vi "SimpleLiveAppWithROI.vi"() -> ()   [LabVIEW 2018]
uses:
  C:/Users/Public/Documents/Photometrics/PMQI-LabViewSamples/Examples/Dependencies/PVCamNET.dll
  Public/Documents/Photometrics/PMQI-LabViewSamples/Examples/Dependencies/PVCamNET.dll
panel:
  in  "Full CCD":bool
  in  "Full CCD Height":u16
  in  "Full CCD Width":u16
  in  "Get ROI":bool
  in  "Height":u16
  in  "Y":u16
  in  "Width":u16
  in  "X":u16
  in  "Exposure Time":dbl
  in  "Live":bool
  in  "Camera Status":bool
  in  "Uninit":bool
  in  "Live stop":bool
  in  "Live start":bool
  in  "Init":bool
  # "SimpleLiveAppWithROI.vi\n\nDescription:\nThis sample code lets the user use live mode in an event driven structure.\nThe user can create a ROI from CamWindow and find out the coordinate.\n\nSteps to run:\n1. Click \"Run\"\n2. Click \"Open\"\n3. Enter Exposure Time\n4. Click \"Live start\"\n5. Click \"Live stop\"\n6. Right click on CamWindow and add a ROI.\n7. Click \"Get ROI\"\n8. Click \"Live start\"\n9. Click \"Live stop\"\n10. Right click on CamWindow and delete a ROI.\n11. Click \"Close\""
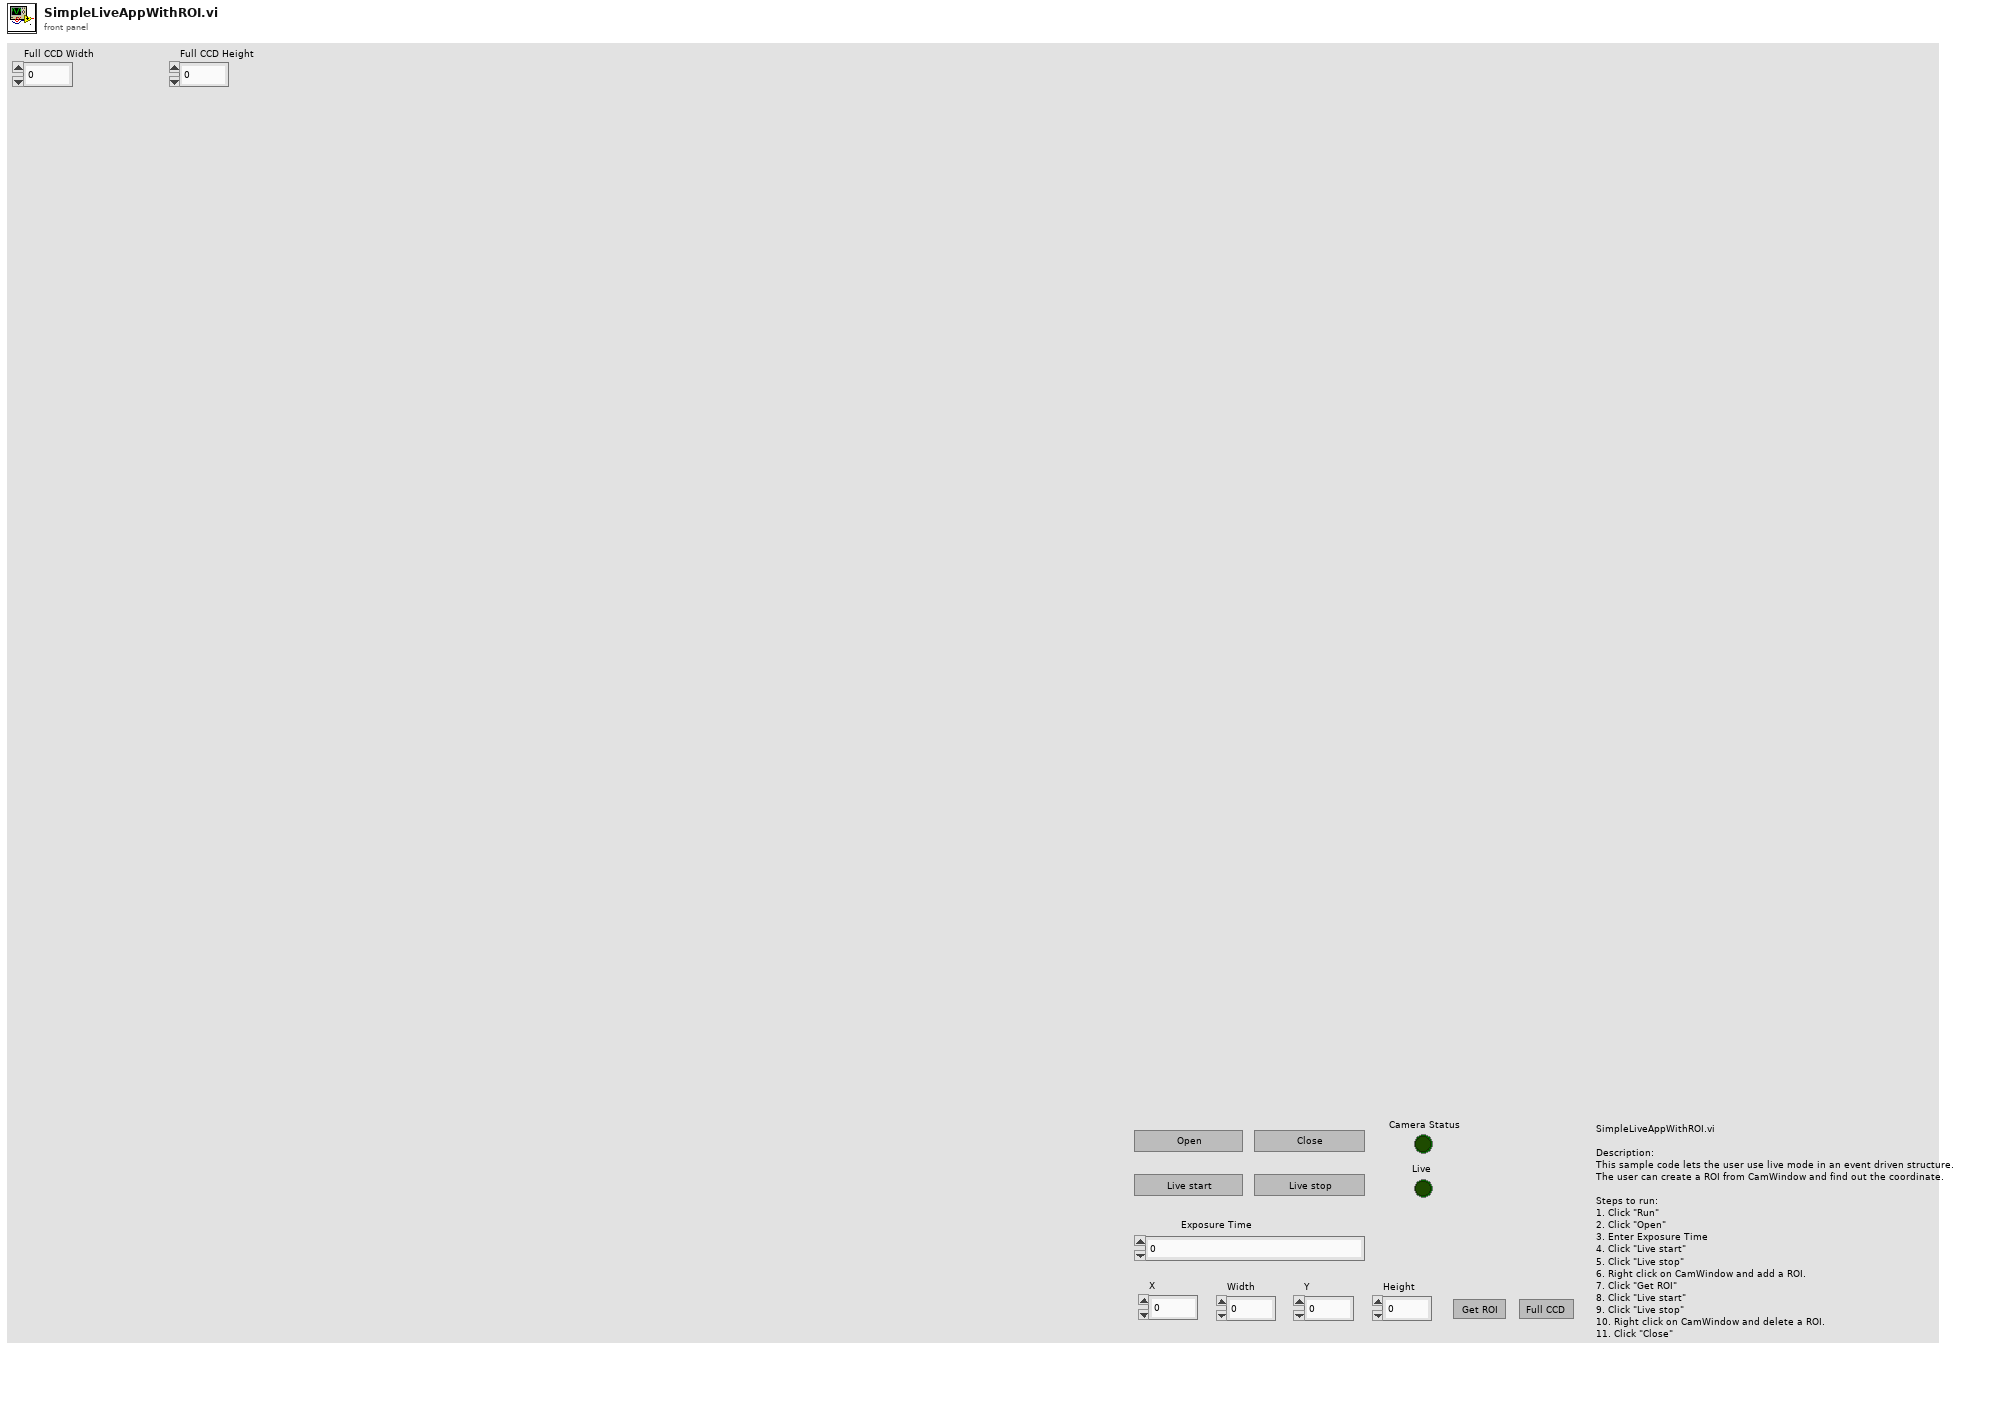
[diagram p1: front panel]
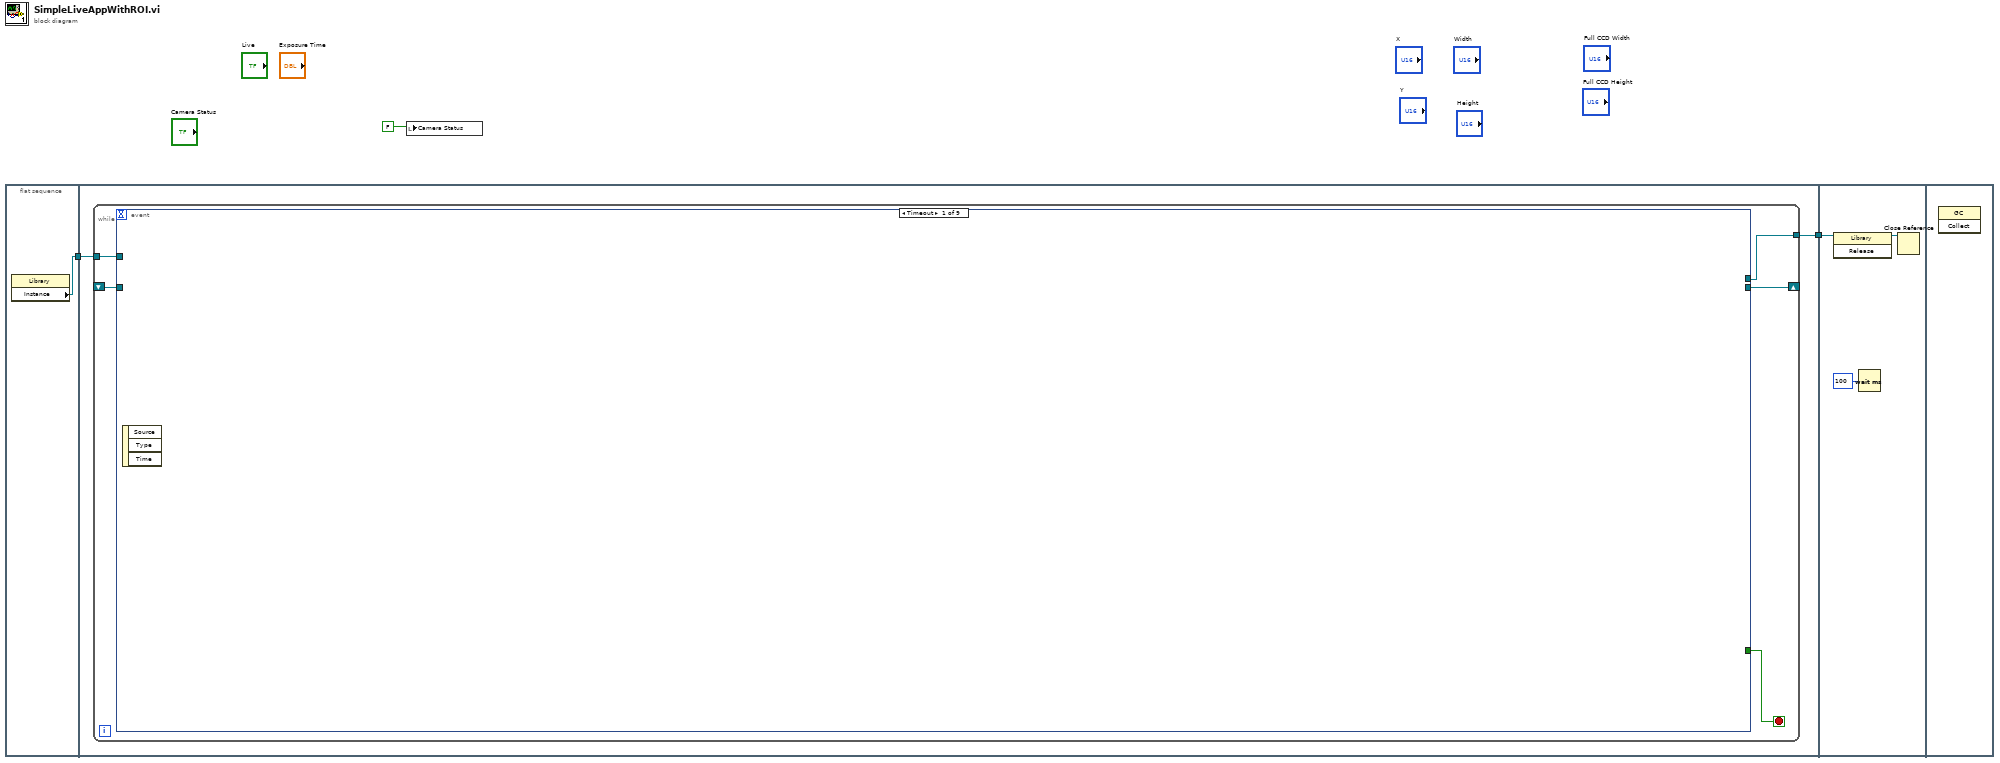
[diagram p0: block diagram]
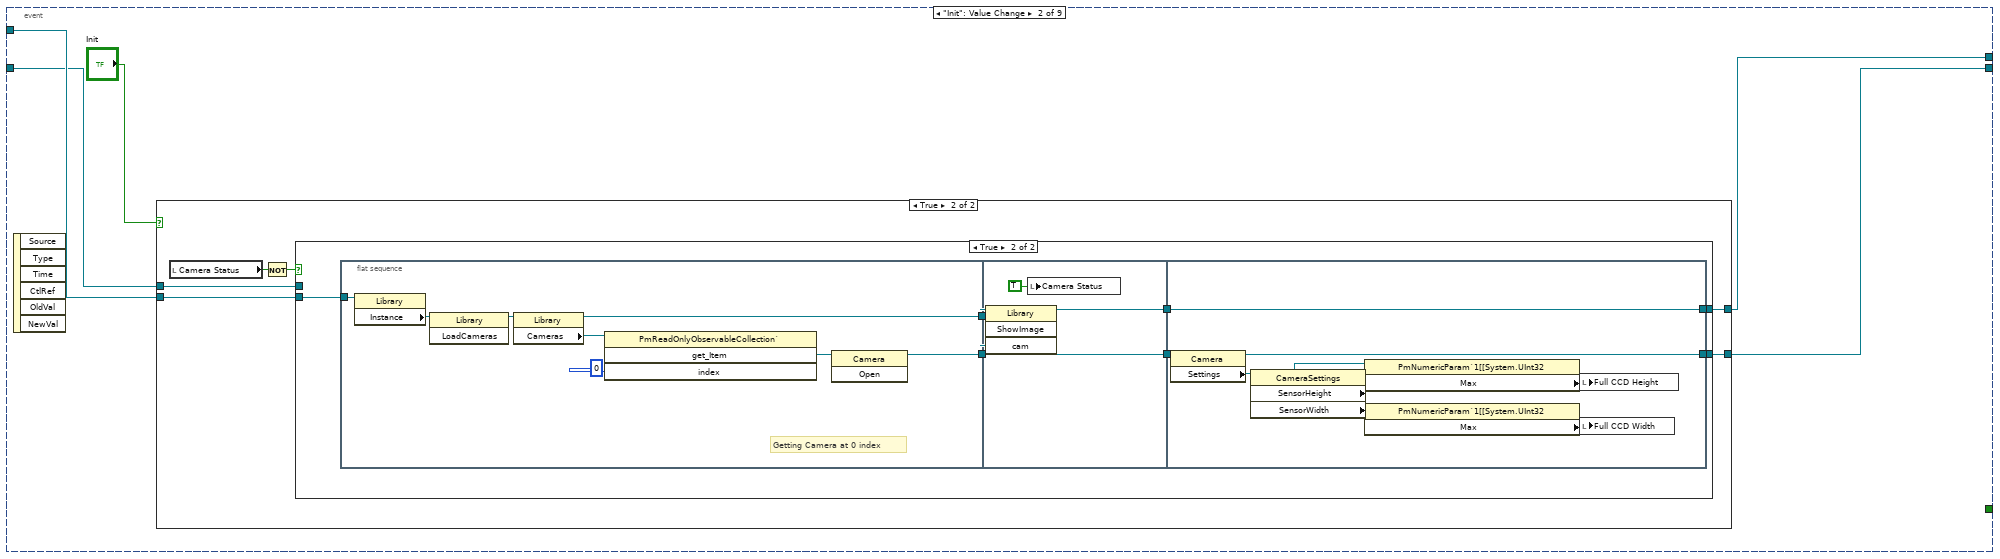
[diagram p2: hidden frame]
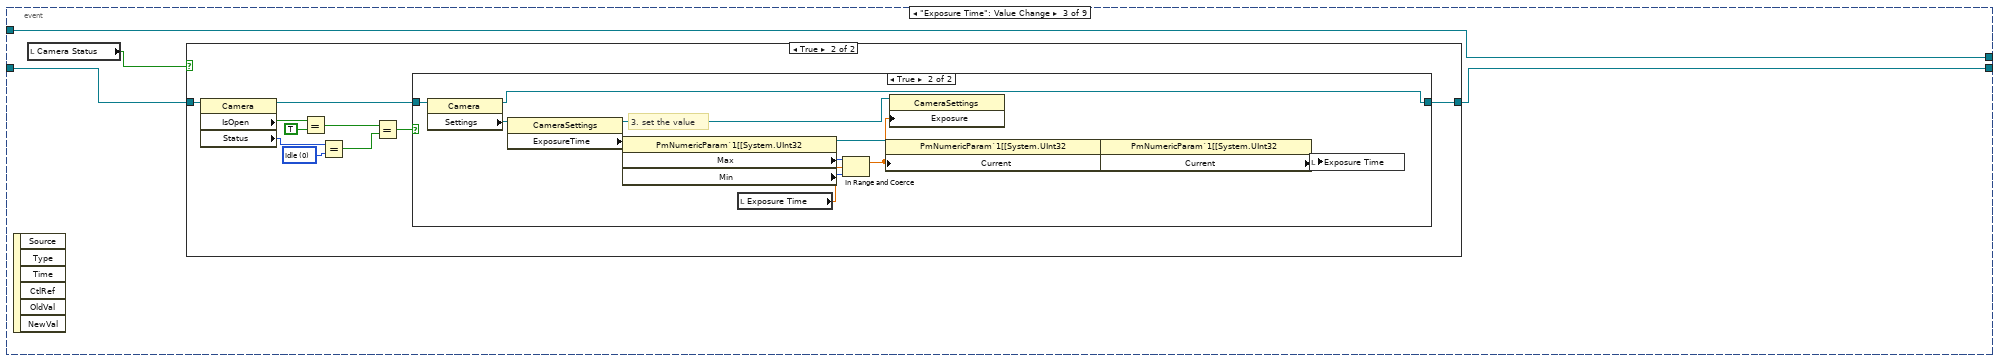
[diagram p5: hidden frame]
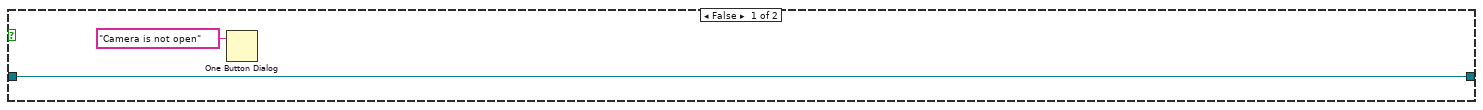
[diagram p6: hidden frame]
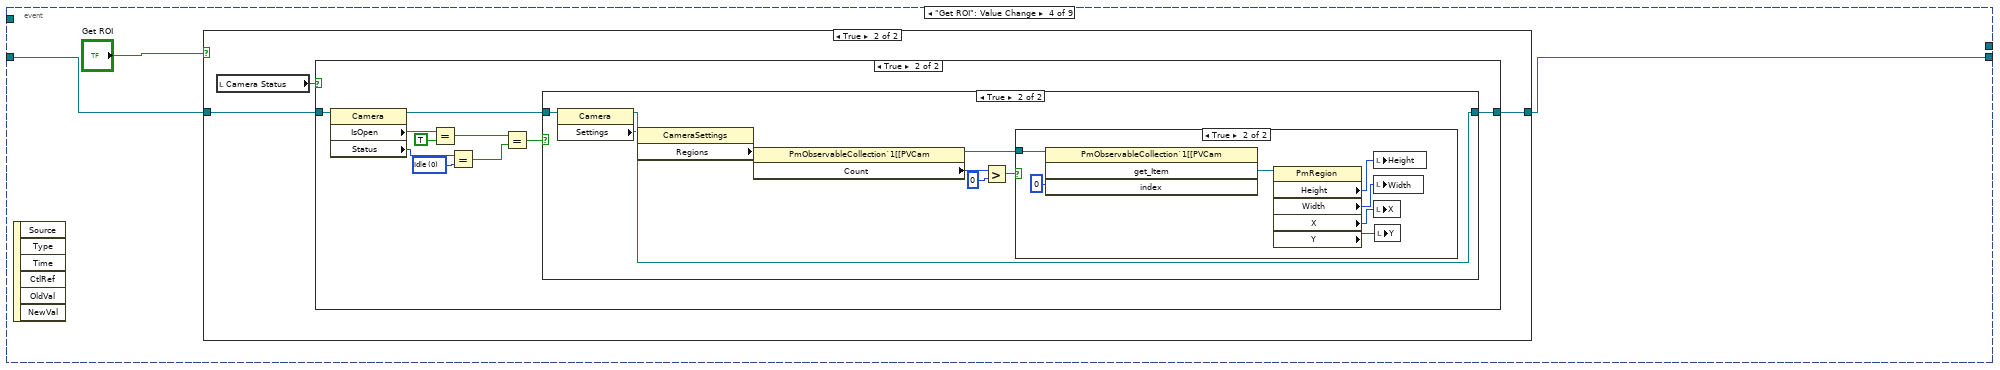
[diagram p8: hidden frame]
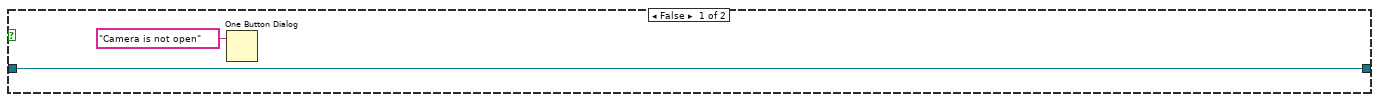
[diagram p10: hidden frame]
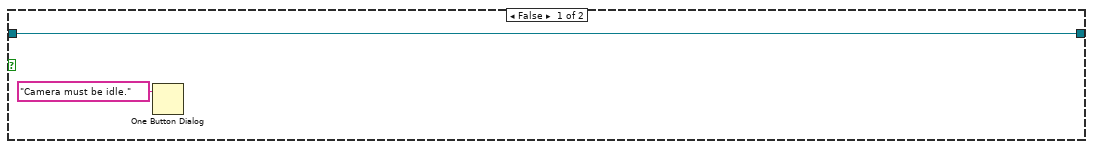
[diagram p11: hidden frame]
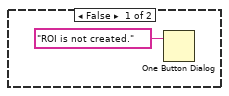
[diagram p12: hidden frame]
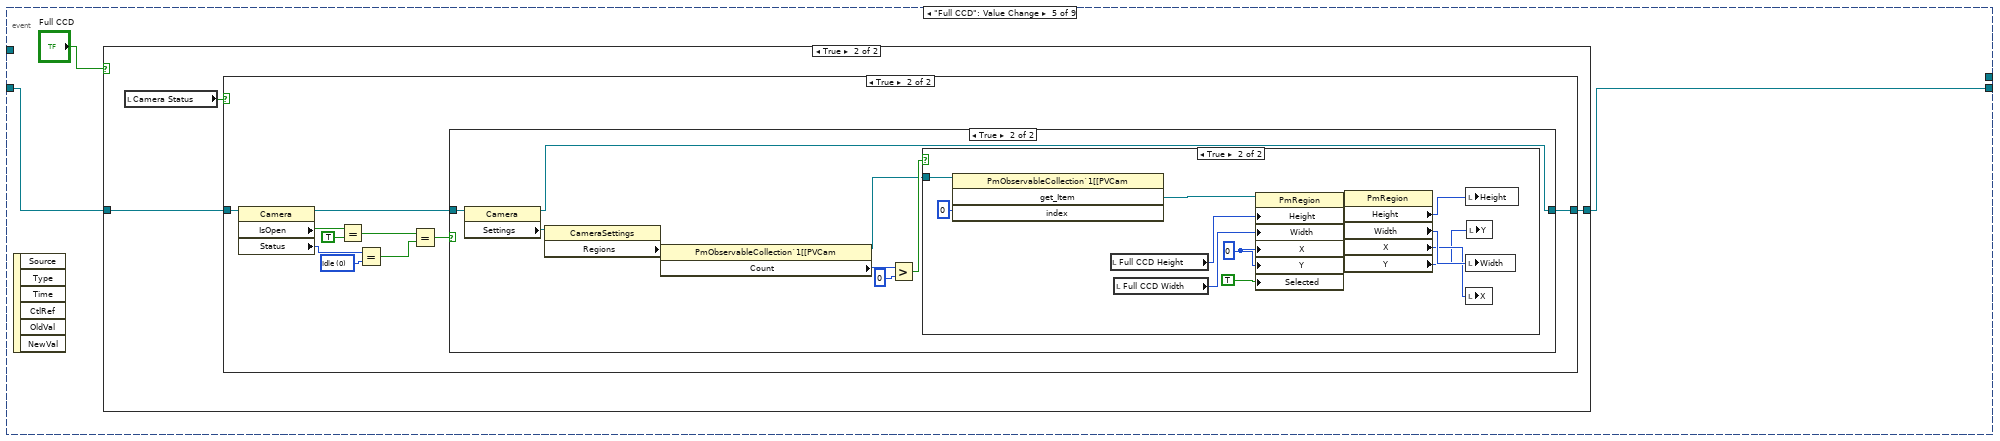
[diagram p13: hidden frame]
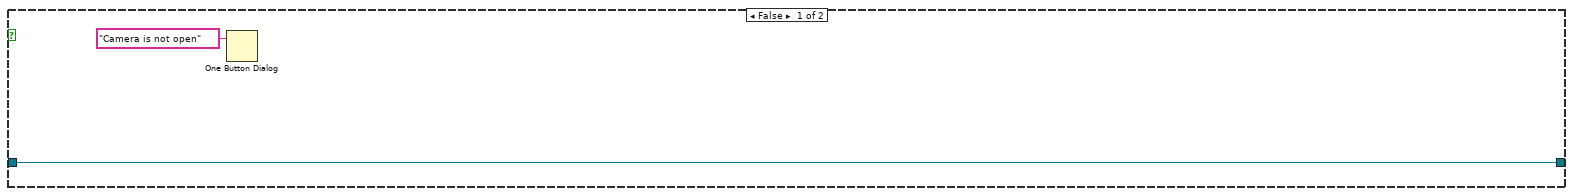
[diagram p15: hidden frame]
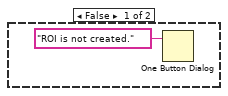
[diagram p17: hidden frame]
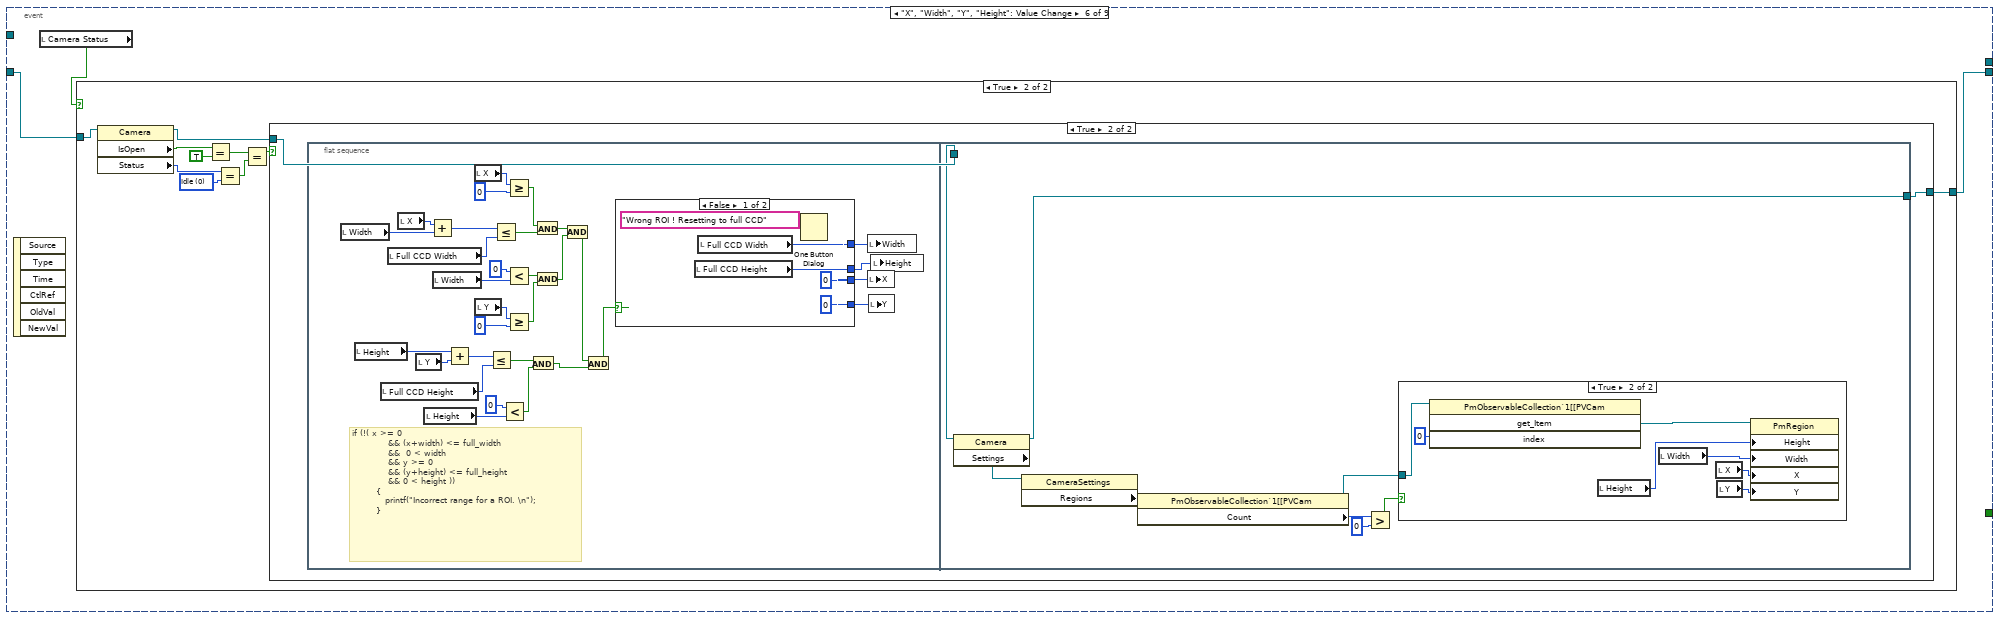
[diagram p18: hidden frame]
diagram:
  n1 = flat-sequence {
    tunnel: [w4] -> w3
    tunnel: w3 -> [w6]
    tunnel: [w5] -> w2
    tunnel: w2 -> [w317]
    frame #0 {
      n2 = property class="Library"() -> ("Instance"=w4:refnum<k24>)  [unwired: 2 in, 2 out]
    }
    frame #1 {
      n3 = while {
        tunnel: w6 -> [w11]
        shift-right: [w7] -> _
        shift-left: _ -> [w9]
        tunnel: [w10] -> w5
        stop <- w8 stop-if-true
        n4 = event shown="[0] Timeout" {
          selector: _ -> [_ _ _ _ _ _ _ _ _]
          dyn-events: _ -> [_ _ _ _ _ _ _ _ _]
          timeout: _ -> [_ _ _ _ _ _ _ _ _]
          tunnel: w11 -> [_ w16 w54 _ _ _ w234 _ w289]
          tunnel: [_ w15 w56 w83 w121 w162 w235 w264 w290] -> w7
          tunnel: [_ w14 w54 _ _ _ w234 _ w289] -> w10
          tunnel: w9 -> [_ w13 w57 w85 w122 w161 w236 w265 w291]
          tunnel: [_ _ _ _ _ _ _ _ w288] -> w8
          event Timeout {
            n5 = event-data() -> ()  [unwired: 1 in, 3 out]
          }
          event "Init": Value Change {
            n6 = event-data() -> ()  [unwired: 1 in, 6 out]
            n7 = case shown="True" "Init" {
              tunnel: w16 -> [w18 w24]
              tunnel: [w17 w23] -> w15
              tunnel: [w18 w22] -> w14
              tunnel: w13 -> [w17 w19]
              frame False {
              }
              frame True {
                n8 = local read "Camera Status"() -> (w21:bool)
                n9 = Not(x=w21) -> (.not. x?=w20:bool)
                n10 = case shown="True" w20 {
                  tunnel: w24 -> [w25 w31]
                  tunnel: [w26 w30] -> w23
                  tunnel: [w25 w29] -> w22
                  tunnel: w19 -> [w26 _]
                  frame False {
                  }
                  frame True {
                    n11 = flat-sequence {
                      tunnel: w31 -> [w36]
                      tunnel: [w38] -> w33
                      tunnel: [w37] -> w32
                      tunnel: w33 -> [w44]
                      tunnel: w32 -> [w45]
                      tunnel: [w45] -> w28
                      tunnel: [w43] -> w27
                      tunnel: [w53] -> w29
                      tunnel: [w48] -> w30
                      tunnel: w28 -> [w52]
                      tunnel: w27 -> [w53]
                      frame #0 {
                        # "Getting Camera at 0 index"
                        n12 = property class="Library"(reference=w36) -> ("Instance"=w35:refnum<k24>)  [unwired: 1 in, 2 out]
                        n13 = invoke class="Library" method="LoadCameras"(reference=w35) -> (reference out=w34:refnum<k24>)  [unwired: 2 in, 2 out]
                        n14 = property class="Library"(reference=w34) -> (reference out=w38:refnum<k24>, "Cameras"=w41:refnum<k24>)  [unwired: 1 in, 1 out]
                        n15 = invoke class="PmReadOnlyObservableCollection`" method="get_Item"(reference=w41, "index"=0) -> ("get_Item"=w39:refnum<k24>)  [unwired: 2 in, 3 out]
                        n16 = invoke class="Camera" method="Open"(reference=w39) -> (reference out=w37:refnum<k24>)  [unwired: 2 in, 2 out]
                      }
                      frame #1 {
                        n17 = invoke class="Library" method="ShowImage"(reference=w44, "cam"=w45) -> (reference out=w43:refnum<k24>)  [unwired: 2 in, 3 out]
                        n18 = local write "Camera Status"(TRUE ("Camera Status")) -> ()
                      }
                      frame #2 {
                        n19 = property class="Camera"(reference=w52) -> (reference out=w48:refnum<k24>, "Settings"=w51:refnum<k24>)  [unwired: 1 in, 1 out]
                        n20 = property class="CameraSettings"(reference=w51) -> ("SensorHeight"=w50:refnum<k24>, "SensorWidth"=w49:refnum<k24>)  [unwired: 1 in, 2 out]
                        n21 = property class="PmNumericParam`1[[System.UInt32"(reference=w50) -> ("Max"=w47:u32)  [unwired: 1 in, 2 out]
                        n22 = property class="PmNumericParam`1[[System.UInt32"(reference=w49) -> ("Max"=w46:u32)  [unwired: 1 in, 2 out]
                        n23 = local write "Full CCD Height"(w47) -> ()
                        n24 = local write "Full CCD Width"(w46) -> ()
                      }
                    }
                  }
                }
              }
            }
          }
          event "Exposure Time": Value Change {
            n25 = event-data() -> ()  [unwired: 1 in, 6 out]
            n26 = local read "Camera Status"() -> (w55:bool)
            n27 = case shown="True" w55 {
              tunnel: w57 -> [w59 w63]
              tunnel: [w59 w60] -> w56
              frame False {
                n28 = One Button Dialog(message="Camera is not open") -> ()  [unwired: 1 in, 1 out]
              }
              frame True {
                w68 = 0 items=["Idle", "Capturing"] ("Status")
                n29 = property class="Camera"(reference=w63) -> (reference out=w61:refnum<k24>, "IsOpen"=w67:bool, "Status"=w69:i32)  [unwired: 1 in, 1 out]
                n30 = Equal?(x=w67, y=TRUE) -> (x = y?=w65:bool)
                n31 = Equal?(x=w69, y=w68) -> (x = y?=w64:bool)
                n32 = Equal?(x=w65, y=w64) -> (x = y?=w62:bool)
                n33 = case shown="True" w62 {
                  tunnel: w61 -> [w70 w82]
                  tunnel: [w70 w71] -> w60
                  frame False {
                  }
                  frame True {
                    # "3. set the value"
                    n34 = property class="Camera"(reference=w82) -> (reference out=w71:refnum<k24>, "Settings"=w81:refnum<k24>)  [unwired: 1 in, 1 out]
                    n35 = property class="CameraSettings"(reference=w81) -> (reference out=w74:refnum<k24>, "ExposureTime"=w75:refnum<k24>)  [unwired: 1 in, 1 out]
                    n36 = property class="PmNumericParam`1[[System.UInt32"(reference=w75) -> (reference out=w78:refnum<k24>, "Max"=w80:u32, "Min"=w79:u32)  [unwired: 1 in, 1 out]
                    n37 = local read "Exposure Time"() -> (w73:dbl)
                    n38 = In Range and Coerce(upper limit=w80, x=w73, lower limit=w79) -> (coerced(x)=w76:dbl)  [unwired: 1 out]
                    n39 = property class="PmNumericParam`1[[System.UInt32"(reference=w78, "Current"=w76) -> (reference out=w77:refnum<k24>)  [unwired: 1 in, 1 out]
                    n40 = property class="CameraSettings"(reference=w74, "Exposure"=w76) -> ()  [unwired: 1 in, 2 out]
                    n41 = property class="PmNumericParam`1[[System.UInt32"(reference=w77) -> ("Current"=w72:u32)  [unwired: 1 in, 2 out]
                    n42 = local write "Exposure Time"(w72) -> ()
                  }
                }
              }
            }
          }
          event "Get ROI": Value Change {
            n43 = event-data() -> ()  [unwired: 1 in, 6 out]
            n44 = case shown="True" "Get ROI" {
              tunnel: w85 -> [w86 w89]
              tunnel: [w86 w88] -> w83
              frame False {
              }
              frame True {
                n45 = local read "Camera Status"() -> (w87:bool)
                n46 = case shown="True" w87 {
                  tunnel: w89 -> [w91 w95]
                  tunnel: [w91 w92] -> w88
                  frame False {
                    n47 = One Button Dialog(message="Camera is not open") -> ()  [unwired: 1 in, 1 out]
                  }
                  frame True {
                    w100 = 0 items=["Idle", "Capturing"] ("Status")
                    n48 = property class="Camera"(reference=w95) -> (reference out=w94:refnum<k24>, "IsOpen"=w99:bool, "Status"=w101:i32)  [unwired: 1 in, 1 out]
                    n49 = Equal?(x=w99, y=TRUE) -> (x = y?=w97:bool)
                    n50 = Equal?(x=w101, y=w100) -> (x = y?=w96:bool)
                    n51 = Equal?(x=w97, y=w96) -> (x = y?=w93:bool)
                    n52 = case shown="True" w93 {
                      tunnel: w94 -> [w103 w111]
                      tunnel: [w103 w110] -> w92
                      frame False {
                        n53 = One Button Dialog(message="Camera must be idle.") -> ()  [unwired: 1 in, 1 out]
                      }
                      frame True {
                        n54 = property class="Camera"(reference=w111) -> (reference out=w110:refnum<k24>, "Settings"=w109:refnum<k24>)  [unwired: 1 in, 1 out]
                        n55 = property class="CameraSettings"(reference=w109) -> ("Regions"=w108:refnum<k24>)  [unwired: 1 in, 2 out]
                        n56 = property class="PmObservableCollection`1[[PVCam"(reference=w108) -> (reference out=w104:refnum<k24>, "Count"=w107:i32)  [unwired: 1 in, 1 out]
                        n57 = Greater?(x=w107, y=0) -> (0:w105:bool)
                        n58 = case shown="True" w105 {
                          tunnel: w104 -> [_ w113]
                          frame False {
                            n59 = One Button Dialog(message="ROI is not created.") -> ()  [unwired: 1 in, 1 out]
                          }
                          frame True {
                            n60 = invoke class="PmObservableCollection`1[[PVCam" method="get_Item"(reference=w113, "index"=0) -> ("get_Item"=w119:refnum<k24>)  [unwired: 2 in, 3 out]
                            n61 = property class="PmRegion"(reference=w119) -> ("Height"=w117:u16, "Width"=w116:u16, "X"=w115:u16, "Y"=w114:u16)  [unwired: 1 in, 2 out]
                            n62 = local write "Height"(w117) -> ()
                            n63 = local write "Width"(w116) -> ()
                            n64 = local write "X"(w115) -> ()
                            n65 = local write "Y"(w114) -> ()
                          }
                        }
                      }
                    }
                  }
                }
              }
            }
          }
          event "Full CCD": Value Change {
            n66 = event-data() -> ()  [unwired: 1 in, 6 out]
            n67 = case shown="True" "Full CCD" {
              tunnel: w122 -> [w123 w126]
              tunnel: [w123 w125] -> w121
              frame False {
              }
              frame True {
                n68 = local read "Camera Status"() -> (w124:bool)
                n69 = case shown="True" w124 {
                  tunnel: w126 -> [w128 w132]
                  tunnel: [w128 w129] -> w125
                  frame False {
                    n70 = One Button Dialog(message="Camera is not open") -> ()  [unwired: 1 in, 1 out]
                  }
                  frame True {
                    w137 = 0 items=["Idle", "Capturing"] ("Status")
                    n71 = property class="Camera"(reference=w132) -> (reference out=w131:refnum<k24>, "IsOpen"=w136:bool, "Status"=w138:i32)  [unwired: 1 in, 1 out]
                    n72 = Equal?(x=w136, y=TRUE) -> (x = y?=w134:bool)
                    n73 = Equal?(x=w138, y=w137) -> (x = y?=w133:bool)
                    n74 = Equal?(x=w134, y=w133) -> (x = y?=w130:bool)
                    n75 = case shown="True" w130 {
                      tunnel: w131 -> [w139 w147]
                      tunnel: [w139 w146] -> w129
                      frame False {
                      }
                      frame True {
                        n76 = property class="Camera"(reference=w147) -> (reference out=w146:refnum<k24>, "Settings"=w145:refnum<k24>)  [unwired: 1 in, 1 out]
                        n77 = property class="CameraSettings"(reference=w145) -> ("Regions"=w144:refnum<k24>)  [unwired: 1 in, 2 out]
                        n78 = property class="PmObservableCollection`1[[PVCam"(reference=w144) -> (reference out=w140:refnum<k24>, "Count"=w143:i32)  [unwired: 1 in, 1 out]
                        n79 = Greater?(x=w143, y=0) -> (0:w141:bool)
                        n80 = case shown="True" w141 {
                          tunnel: w140 -> [_ w158]
                          frame False {
                            n81 = One Button Dialog(message="ROI is not created.") -> ()  [unwired: 1 in, 1 out]
                          }
                          frame True {
                            w149 = u16 0 ("X")
                            n82 = invoke class="PmObservableCollection`1[[PVCam" method="get_Item"(reference=w158, "index"=0) -> ("get_Item"=w160:refnum<k24>)  [unwired: 2 in, 3 out]
                            n83 = local read "Full CCD Height"() -> (w155:u16)
                            n84 = local read "Full CCD Width"() -> (w156:u16)
                            n85 = property class="PmRegion"(reference=w160, "Height"=w155, "Width"=w156, "X"=w149, "Y"=w149, "Selected"=TRUE) -> (reference out=w154:refnum<k24>)  [unwired: 1 in, 1 out]
                            n86 = property class="PmRegion"(reference=w154) -> ("Height"=w153:u16, "Width"=w152:u16, "X"=w151:u16, "Y"=w150:u16)  [unwired: 1 in, 2 out]
                            n87 = local write "Height"(w153) -> ()
                            n88 = local write "Width"(w152) -> ()
                            n89 = local write "X"(w151) -> ()
                            n90 = local write "Y"(w150) -> ()
                          }
                        }
                      }
                    }
                  }
                }
              }
            }
          }
          event "X", "Width", "Y", "Height": Value Change {
            n91 = event-data() -> ()  [unwired: 1 in, 6 out]
            n92 = local read "Camera Status"() -> (w163:bool)
            n93 = case shown="True" w163 {
              tunnel: w161 -> [w164 w167]
              tunnel: [w164 w165] -> w162
              frame False {
              }
              frame True {
                w173 = 0 items=["Idle", "Capturing"] ("Status")
                n94 = property class="Camera"(reference=w167) -> (reference out=w166:refnum<k24>, "IsOpen"=w172:bool, "Status"=w174:i32)  [unwired: 1 in, 1 out]
                n95 = Equal?(x=w172, y=TRUE) -> (x = y?=w170:bool)
                n96 = Equal?(x=w174, y=w173) -> (x = y?=w169:bool)
                n97 = Equal?(x=w170, y=w169) -> (x = y?=w168:bool)
                n98 = case shown="True" w168 {
                  tunnel: w166 -> [w175 w177]
                  tunnel: [w175 w176] -> w165
                  frame False {
                  }
                  frame True {
                    n99 = flat-sequence {
                      tunnel: w177 -> [w225]
                      tunnel: [w224] -> w176
                      frame #0 {
                        # "if (!( x >= 0\n            && (x+width) <= full_width\n            &&  0 < width \n            && y >= 0\n            && (y+height) <= full_height\n            && 0 < height ))\n        {\n           printf(\"Incorrect range for a ROI. \\n\");\n        }"
                        n100 = local read "Width"() -> (w193:u16)
                        n101 = local read "Height"() -> (w191:u16)
                        n102 = local read "Full CCD Height"() -> (w187:u16)
                        n103 = local read "Full CCD Width"() -> (w189:u16)
                        n104 = local read "X"() -> (w194:u16)
                        n105 = local read "Y"() -> (w190:u16)
                        n106 = local read "Height"() -> (w182:u16)
                        n107 = Add(x=w194, y=w193) -> (x+y=w188:u16)
                        n108 = local read "Width"() -> (w185:u16)
                        n109 = Add(x=w191, y=w190) -> (x+y=w186:u16)
                        n110 = local read "X"() -> (w195:u16)
                        n111 = local read "Y"() -> (w192:u16)
                        n112 = Less Or Equal?(x=w186, y=w187) -> (x <= y?=w202:bool)
                        n113 = Less Or Equal?(x=w188, y=w189) -> (x <= y?=w205:bool)
                        n114 = Less?(x=u16 0 ("y"), y=w182) -> (x < y?=w201:bool)
                        n115 = Greater Or Equal?(x=w195, y=u16 0) -> (x >= y?=w206:bool)
                        n116 = Less?(x=u16 0 ("y"), y=w185) -> (x < y?=w204:bool)
                        n117 = Greater Or Equal?(x=w192, y=u16 0) -> (x >= y?=w203:bool)
                        n118 = And(x=w202, y=w201) -> (x .and. y?=w197:bool)
                        n119 = And(x=w206, y=w205) -> (x .and. y?=w200:bool)
                        n120 = And(x=w204, y=w203) -> (x .and. y?=w199:bool)
                        n121 = And(x=w200, y=w199) -> (x .and. y?=w198:bool)
                        n122 = And(x=w198, y=w197) -> (x .and. y?=w196:bool)
                        n123 = case shown="False" w196 {
                          tunnel: [w210 w217] -> w181
                          tunnel: [u16 0 ("X") w216] -> w178
                          tunnel: [u16 0 ("Y") w215] -> w179
                          tunnel: [w211 w214] -> w180
                          frame False {
                            n124 = local read "Full CCD Height"() -> (w211:u16)
                            n125 = local read "Full CCD Width"() -> (w210:u16)
                            n126 = One Button Dialog(message="Wrong ROI ! Resetting to full CCD") -> ()  [unwired: 1 in, 1 out]
                          }
                          frame True {
                            n127 = local read "Height"() -> (w214:u16)
                            n128 = local read "Width"() -> (w217:u16)
                            n129 = local read "X"() -> (w216:u16)
                            n130 = local read "Y"() -> (w215:u16)
                          }
                        }
                        n131 = local write "Width"(w181) -> ()
                        n132 = local write "X"(w178) -> ()
                        n133 = local write "Y"(w179) -> ()
                        n134 = local write "Height"(w180) -> ()
                      }
                      frame #1 {
                        n135 = property class="Camera"(reference=w225) -> (reference out=w224:refnum<k24>, "Settings"=w223:refnum<k24>)  [unwired: 1 in, 1 out]
                        n136 = property class="CameraSettings"(reference=w223) -> ("Regions"=w222:refnum<k24>)  [unwired: 1 in, 2 out]
                        n137 = property class="PmObservableCollection`1[[PVCam"(reference=w222) -> (reference out=w218:refnum<k24>, "Count"=w221:i32)  [unwired: 1 in, 1 out]
                        n138 = Greater?(x=w221, y=0) -> (0:w219:bool)
                        n139 = case shown="True" w219 {
                          tunnel: w218 -> [_ w231]
                          frame False {
                            n140 = One Button Dialog(message="ROI is not created.") -> ()  [unwired: 1 in, 1 out]
                          }
                          frame True {
                            n141 = invoke class="PmObservableCollection`1[[PVCam" method="get_Item"(reference=w231, "index"=0) -> ("get_Item"=w233:refnum<k24>)  [unwired: 2 in, 3 out]
                            n142 = local read "Height"() -> (w230:u16)
                            n143 = local read "Width"() -> (w229:u16)
                            n144 = local read "X"() -> (w228:u16)
                            n145 = local read "Y"() -> (w227:u16)
                            n146 = property class="PmRegion"(reference=w233, "Height"=w230, "Width"=w229, "X"=w228, "Y"=w227) -> ()  [unwired: 1 in, 2 out]
                          }
                        }
                      }
                    }
                  }
                }
              }
            }
          }
          event "Live start": Value Change {
            n147 = event-data() -> ()  [unwired: 1 in, 6 out]
            n148 = case shown="True" "Live start" {
              tunnel: w236 -> [w238 w241]
              tunnel: [w238 w240] -> w235
              frame False {
              }
              frame True {
                n149 = local read "Camera Status"() -> (w239:bool)
                n150 = case shown="True" w239 {
                  tunnel: w241 -> [w242 w247]
                  tunnel: [w242 w245] -> w240
                  frame False {
                    n151 = One Button Dialog(message="Camera is not open") -> ()  [unwired: 1 in, 1 out]
                  }
                  frame True {
                    w252 = 0 items=["Idle", "Capturing"] ("Status")
                    n152 = property class="Camera"(reference=w247) -> (reference out=w246:refnum<k24>, "IsOpen"=w251:bool, "Status"=w253:i32)  [unwired: 1 in, 1 out]
                    n153 = Equal?(x=w251, y=TRUE) -> (x = y?=w249:bool)
                    n154 = Equal?(x=w253, y=w252) -> (x = y?=w248:bool)
                    n155 = Equal?(x=w249, y=w248) -> (x = y?=w244:bool)
                    n156 = case shown="True" w244 {
                      tunnel: w246 -> [w255 w257]
                      tunnel: [w255 w258] -> w245
                      frame False {
                        n157 = local write "Live"(FALSE ("Live 2")) -> ()
                      }
                      frame True {
                        n158 = flat-sequence {
                          tunnel: w257 -> [w263]
                          tunnel: [w260] -> w256
                          frame #0 {
                            n159 = property class="Camera"(reference=w263) -> (reference out=w260:refnum<k24>, "AcquisitionBuffer"=w262:refnum<k24>)  [unwired: 1 in, 1 out]
                            n160 = property class="AcqBuffer"(reference=w262, "BufferSize"=50) -> ()  [unwired: 1 in, 2 out]
                          }
                        }
                        n161 = local write "Live"(TRUE ("Live")) -> ()
                        n162 = invoke class="Camera" method="StartLive"(reference=w256) -> (reference out=w258:refnum<k24>)  [unwired: 2 in, 2 out]
                      }
                    }
                  }
                }
              }
            }
          }
          event "Live stop": Value Change {
            n163 = event-data() -> ()  [unwired: 1 in, 6 out]
            n164 = case shown="True" "Live stop" {
              tunnel: w265 -> [w267 w270]
              tunnel: [w267 w269] -> w264
              frame False {
              }
              frame True {
                n165 = local read "Camera Status"() -> (w268:bool)
                n166 = case shown="False" w268 {
                  tunnel: w270 -> [w272 w282]
                  tunnel: [w272 w279] -> w269
                  frame False {
                    n167 = One Button Dialog(message="Camera is not open") -> ()  [unwired: 1 in, 1 out]
                  }
                  frame True {
                    w277 = 1 items=["Idle", "Capturing"] ("Status")
                    n168 = property class="Camera"(reference=w282) -> (reference out=w280:refnum<k24>, "IsOpen"=w276:bool, "Status"=w278:i32)  [unwired: 1 in, 1 out]
                    n169 = Equal?(x=w278, y=w277) -> (x = y?=w273:bool)
                    n170 = Equal?(x=w276, y=TRUE) -> (x = y?=w274:bool)
                    n171 = Equal?(x=w274, y=w273) -> (x = y?=w281:bool)
                    n172 = case shown="True" w281 {
                      tunnel: w280 -> [w283 w286]
                      tunnel: [w283 w285] -> w279
                      frame False {
                      }
                      frame True {
                        n173 = invoke class="Camera" method="Stop"(reference=w286) -> (reference out=w285:refnum<k24>)  [unwired: 2 in, 2 out]
                        n174 = local write "Live"(FALSE ("Live 2")) -> ()
                      }
                    }
                  }
                }
              }
            }
          }
          event "Uninit": Value Change {
            n175 = event-data() -> ()  [unwired: 1 in, 6 out]
            n176 = case shown="True" "Uninit" {
              tunnel: w291 -> [w293 w297]
              tunnel: [w293 w296] -> w290
              tunnel: [FALSE ("Camera Status") w294] -> w288
              frame False {
              }
              frame True {
                n177 = local read "Camera Status"() -> (w295:bool)
                n178 = case shown="True" w295 {
                  tunnel: w297 -> [w299 w304]
                  tunnel: [w299 w303] -> w296
                  tunnel: [FALSE ("Camera Status") w302] -> w294
                  frame False {
                  }
                  frame True {
                    n179 = local read "Live"() -> (w300:bool)
                    n180 = Not(x=w300) -> (.not. x?=w301:bool)
                    n181 = case shown="True" w301 {
                      tunnel: w304 -> [w306 w309]
                      tunnel: [w306 w308] -> w303
                      tunnel: [FALSE ("Camera Status") w307] -> w302
                      frame False {
                      }
                      frame True {
                        n182 = flat-sequence {
                          tunnel: w309 -> [w312]
                          tunnel: [w311] -> w310
                          tunnel: [w315] -> w308
                          tunnel: w310 -> [w315]
                          tunnel: [TRUE ("Camera Status")] -> w307
                          frame #0 {
                            n183 = invoke class="Camera" method="Close"(reference=w312) -> (reference out=w311:refnum<k24>)  [unwired: 2 in, 2 out]
                          }
                          frame #1 {
                            n184 = local write "Camera Status"(FALSE ("Camera Status")) -> ()
                          }
                        }
                      }
                    }
                  }
                }
              }
            }
          }
        }
      }
    }
    frame #2 {
      n185 = invoke class="Library" method="Release"(reference=w317) -> (reference out=w318:refnum<k24>)  [unwired: 2 in, 2 out]
      n186 = Wait (ms)(milliseconds to wait=u32 100) -> ()  [unwired: 1 out]
      n187 = Close Reference(reference=w318) -> ()  [unwired: 1 in, 1 out]
    }
    frame #3 {
      n188 = invoke class="GC" method="Collect"() -> ()  [unwired: 3 in, 3 out]
    }
  }
  n189 = local write "Camera Status"(FALSE ("Camera Status")) -> ()
